vi "GEA2_OR_GEA3.vi"(0 "session in":refnum<k35>, 2 "board":u8, 11 "error in (no error)":errorcluster) -> (4 "session out":refnum<k35>, 8 "GEA":string, 15 "error out":errorcluster)   [LabVIEW 2021]
panel:
  out "Raw Data":string
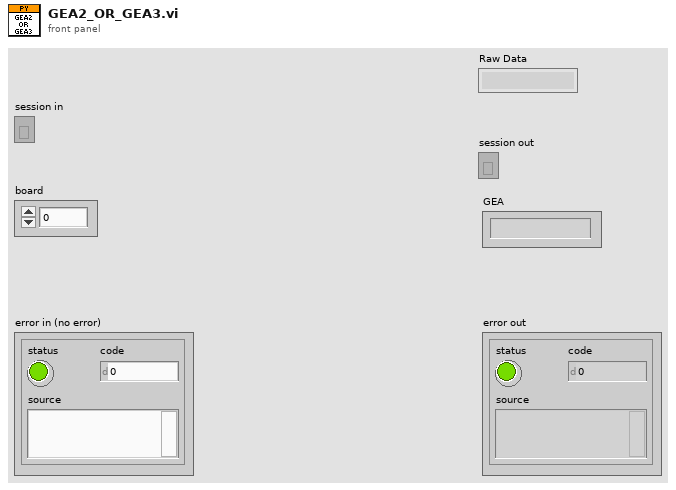
[diagram p1: front panel]
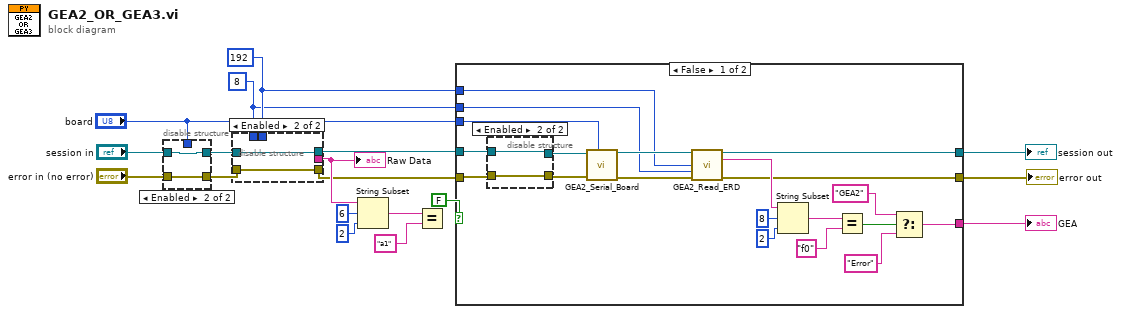
[diagram p0: block diagram]
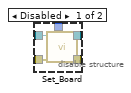
[diagram p2: hidden frame]
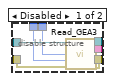
[diagram p3: hidden frame]
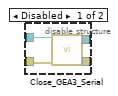
[diagram p4: hidden frame]
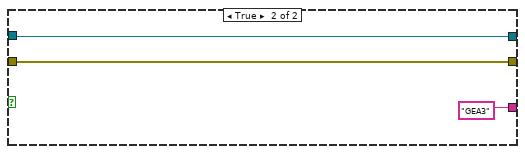
[diagram p5: hidden frame]
diagram:
  w8 = i64 192 ("dst")
  w7 = i64 8 ("ERD")
  n1 = disable-structure shown="Enabled" {
    disable-tunnel: [w23 w25] -> w18
    disable-tunnel: [w22 w24] -> w17
    disable-tunnel: "board" -> [w21 _]
    disable-tunnel: "session in" -> [w20 w25]
    disable-tunnel: "error in (no error)" -> [w19 w24]
    frame Disabled {
      n2 = call "Set_Board.vi"("Board"=w21, "error in (no error)"=w19, "session in"=w20) -> ("error out"=w22:errorcluster, "session out"=w23:refnum<k35>)  [unwired: 7 in]
    }
    frame Enabled {
    }
  }
  n3 = disable-structure shown="Enabled" {
    disable-tunnel: w18 -> [w32 w34]
    disable-tunnel: w17 -> [w31 w33]
    disable-tunnel: [w30 _] -> w16
    disable-tunnel: [w29 w34] -> w11
    disable-tunnel: [w28 w33] -> w10
    disable-tunnel: w8 -> [w27 _]
    disable-tunnel: w7 -> [w26 _]
    frame Disabled {
      n4 = call "Read_GEA3.vi"("session in"=w32, "dst"=w27, "ERD"=w26, "error in (no error)"=w31) -> ("session out"=w29:refnum<k35>, "Raw Data"=w30:string, "error out"=w28:errorcluster)  [unwired: 8 in, 1 out]
    }
    frame Enabled {
    }
  }
  "Raw Data" <- w16
  n5 = String Subset(string=w16, offset (0)=6, length (rest)=2 ("length (rest)")) -> (substring=w13:string)
  n6 = Equal?(x=w13, y="a1") -> ()  [unwired: 1 out]
  n7 = case shown="False" FALSE {
    tunnel: [w41 "GEA3"] -> w6
    tunnel: w11 -> [w40 w62]
    tunnel: w10 -> [w38 w61]
    tunnel: "board" -> [w52 _]
    tunnel: w8 -> [w51 _]
    tunnel: w7 -> [w50 _]
    tunnel: [w36 w61] -> w2
    tunnel: [w35 w62] -> w3
    frame False {
      n8 = disable-structure shown="Enabled" {
        disable-tunnel: w40 -> [w58 w60]
        disable-tunnel: [w57 w60] -> w39
        disable-tunnel: w38 -> [w56 w59]
        disable-tunnel: [w55 w59] -> w37
        frame Disabled {
          n9 = call "Close_GEA3_Serial.vi"("session in"=w58, "error in (no error)"=w56) -> ("session out"=w57:refnum<k35>, "error out"=w55:errorcluster)  [unwired: 12 in]
        }
        frame Enabled {
        }
      }
      n10 = call "GEA2_Serial_Board.vi"("Board"=w52, "error in (no error)"=w37, "session in"=w39) -> ("error out"=w53:errorcluster, "session out"=w54:refnum<k35>)  [unwired: 7 in]
      n11 = call "GEA2_Read_ERD.vi"("session in"=w54, "dst"=w51, "ERD"=w50, "error in (no error)"=w53) -> ("session out"=w35:refnum<k35>, "Raw Data"=w45:string, "error out"=w36:errorcluster)  [unwired: 8 in, 1 out]
      n12 = String Subset(string=w45, offset (0)=8, length (rest)=2 ("length (rest)")) -> (substring=w47:string)
      n13 = Equal?(x=w47, y="f0") -> (x = y?=w44:bool)
      n14 = Select(t="GEA2", s=w44, f="Error") -> (s? t:f=w41:string)
    }
    frame True {
    }
  }
  "GEA" <- w6
  "session out" <- w3
  "error out" <- w2
